vi "Teleop.vi"(10 "Match Info":T1={"Autonomous Elapsed Seconds"=0.0, "TeleOp Elapsed Seconds"=0.0, "Disabled Elapsed Seconds"=0.0, "Visited Autonomous"=FALSE, "Visited TeleOp"=FALSE, "Visited Disabled"=FALSE, "Autonomous Settings"={"Autonomous Style"=enum."Independent", "VI Refnum"=refnum}}, 11 "Call Context":T2) -> ()   [LabVIEW 2012]
doc: "This VI is called for each TeleOp packet received from the DS where the robot is not disabled. It is often used to read from the joysticks and update I/O or to update setpoints for timed control loops. It should complete and return within 20 milliseconds or it may miss DS packets."
uses:
  <vilib>/Rock Robotics/WPI/DriverStation/WPI_DriverStationDerivedRobotMode.ctl
  <vilib>/Rock Robotics/WPI/DriverStation/WPI_DriverStationMatch Info.ctl
  <vilib>/Rock Robotics/WPI/CAN/Jaguar/SubVIs/WPI_CANJaguar_StatusSelect.ctl
  <vilib>/Rock Robotics/WPI/DriverStation/DriverStationLCD/WPI_DriverStationLCDLCDLine.ctl
  <vilib>/Rock Robotics/WPI/Relay/WPI_RelayValue.ctl
  Robot Global Data.vi
  <vilib>/Rock Robotics/WPI/Joystick/WPI_JoystickGetSetRefNum.vi
  <vilib>/Rock Robotics/WPI/CAN/Jaguar/SubVIs/WPI_CANJaguar_StatusChannelSelect.ctl
  <vilib>/Rock Robotics/WPI/RobotDrive/WPI_RobotDriveMecanumDrive_Cartesian.vi
panel:
  in  "ShooterSpeed":dbl=1000.0
  in  "BallScrewPosition":dbl=0.55
  in  "Position":dbl
  # "KEEP BETWEEN 0.5 AND 0.6"
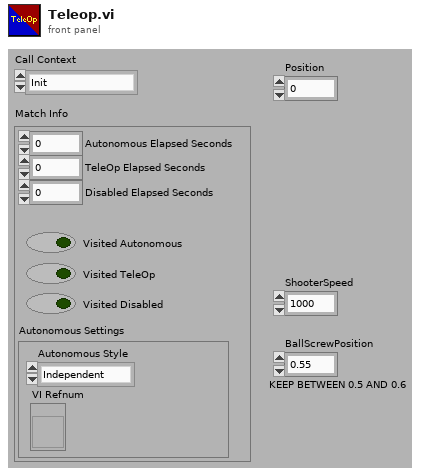
[diagram p1: front panel]
types:
  T1 = typedef "WPI_DriverStationMatch Info.ctl" = cluster{"Autonomous Elapsed Seconds":dbl, "TeleOp Elapsed Seconds":dbl, "Disabled Elapsed Seconds":dbl, "Visited Autonomous":bool, "Visited TeleOp":bool, "Visited Disabled":bool, "Autonomous Settings":cluster{"Autonomous Style":enum16{"Iterative", "Independent"}, "VI Refnum":refnum<vi>}}
  T2 = typedef "WPI_DriverStationDerivedRobotMode.ctl" = enum16{"Init", "Execute", "Stop"}
  T3 = typedef "WPI_DriverStationLCDLCDLine.ctl" = enum16{"Main - Line 1", "User - Line 2", "User - Line 3", "User - Line 4", "User - Line 5", "User - Line 6"}
  T4 = typedef "WPI_CANJaguar_StatusSelect.ctl" = enum16{"Output Percent VBus", "Output Voltage", "Bus Voltage", "Current", "Temperature", "Position", "Speed", "Limit Switches", "Faults", "Fault Counters", "Power Cycle"}
  T5 = cluster{bool, bool, bool, bool, bool, bool, i32, i32}
  T6 = typedef "WPI_JoystickDevRef.ctl" = cluster{"Device":T7}
  T7 = typedef "WPI_JoystickDeviceEnum.ctl" = enum16{"USB 1", "USB 2", "USB 3", "USB 4", "Kinect 1", "Kinect 2"}
  T8 = typedef "WPI_MotorControlDeviceRef.ctl" = cluster{"DeviceStatus":errorcluster, "Type":enum16{"PWM", "CAN"}, "PWM":cluster{"Digital Module":T9, "PWM Channel":T10, "DeadBand":T11}, "CAN":cluster{"Device Number":u8, "Control Mode":T12, "Semaphore":T13, "Max Vout":dbl}, "Invert":bool, "TransformRef":T14, "InvTransformRef":T14}
  T9 = typedef "FPGA_TypedefDigitalModule.ctl" = enum16{"Digital Module 1", "Digital Module 2"}
  T10 = typedef "FPGA_DIOPWMChannel.ctl" = enum8{"PWM 1", "PWM 2", "PWM 3", "PWM 4", "PWM 5", "PWM 6", "PWM 7", "PWM 8", "PWM 9", "PWM 10", "Invalid"}
  T11 = typedef "WPI_PWMDeadband.ctl" = cluster{"Name":string, "maxPositivePwm":i32, "minPositivePwm":i32, "centerPwm":i32, "maxNegativePwm":i32, "minNegativePwm":i32, "angularRange":u16}
  T12 = typedef "WPI_CANJaguar_ControlMode.ctl" = enum8{"Percent VBus", "Current", "Speed", "Position", "Voltage"}
  T13 = typedef "Semaphore RefNum" = refnum<k1>
  T14 = typedef "WPI_PWMTransform_ConPane.ctl" = refnum<vi>
  T15 = cluster{"Position":cluster{"X":dbl, "Y":dbl}, "Distance (ft)":dbl}
  T16 = typedef "WPI_DigitalInputDevRef.ctl" = cluster{"DevStatus":errorcluster, "DIO Channel":T17, "Digital Module":T9}
  T17 = typedef "FPGA_DIOChannel.ctl" = enum8{"DIO 1", "DIO 2", "DIO 3", "DIO 4", "DIO 5", "DIO 6", "DIO 7", "DIO 8", "DIO 9", "DIO 10", "DIO 11", "DIO 12", "DIO 13", "DIO 14", "Invalid"}
  T18 = typedef "WPI_RelayDevRef.ctl" = cluster{"DevStatus":errorcluster, "Relay Channel":T19, "Digital Module":T9, "Relay Direction":T20}
  T19 = typedef "FPGA_DIORelayChannel.ctl" = enum8{"Relay 1", "Relay 2", "Relay 3", "Relay 4", "Relay 5", "Relay 6", "Relay 7", "Relay 8", "Invalid"}
  T20 = typedef "WPI_RelayDirection.ctl" = enum16{"Both directions", "Forward only", "Reverse only"}
  T21 = typedef "WPI_CANJaguar_Status.ctl" = cluster{"Output Percent VBus":dbl, "Output Voltage":dbl, "Bus Voltage":dbl, "Current":dbl, "Temperature":dbl, "Position":dbl, "Speed":dbl, "Limits":cluster{"Forward Limit":bool, "Reverse Limit":bool, "Forward Soft Limit":bool, "Reverse Soft Limit":bool, "Sticky Forward Limit":bool, "Sticky Reverse Limit":bool, "Sticky Forward Soft Limit":bool, "Sticky Reverse Soft Limit":bool}, "Faults":cluster{"Current Fault":bool, "Temperature Fault":bool, "Bus Voltage Fault":bool, "Gate Driver Fault":bool, "Comm Fault":bool}, "Fault Counters":cluster{"Current Faults":u8, "Temperature Faults":u8, "Bus Voltage Faults":u8, "Gate Driver Faults":u8, "Comm Faults":u8, "CAN Status":u8, "CAN RX Errors":u8, "CAN TX Errors":u8}, "Power Cycle":bool}
  T22 = typedef "WPI_JoystickButtonState.ctl" = cluster{"Button 1":bool, "Button 2":bool, "Button 3":bool, "Button 4":bool, "Button 5":bool, "Button 6":bool, "Button 7":bool, "Button 8":bool, "Button 9":bool, "Button 10":bool, "Button 11":bool, "Button 12":bool}
  T23 = typedef "WPI_RelayValue.ctl" = enum16{"Off", "On", "Forward", "Reverse"}
  T24 = cluster{"axis 1 (x)":dbl, "axis 2 (y)":dbl, "axis 3 (throttle)":dbl, "axis 4":dbl, "axis 5":dbl, "axis 6":dbl}
  T25 = typedef "WPI_RobotDriveDevRef.ctl" = cluster{"DevStatus":errorcluster, "Motors[]":T8[], "Square Inputs":bool, "Max Output":dbl, "Isochronous":bool}
  T26 = typedef "WPI_CANJaguar_StatusChannelSelect.ctl" = enum16{"Periodic Status Channel 1", "Periodic Status Channel 2", "Periodic Status Channel 3", "Periodic Status Channel 4", "On Demand Status"}
  T27 = cluster{bool, bool, bool, bool, bool, bool, "DistanceOut":dbl, i32}
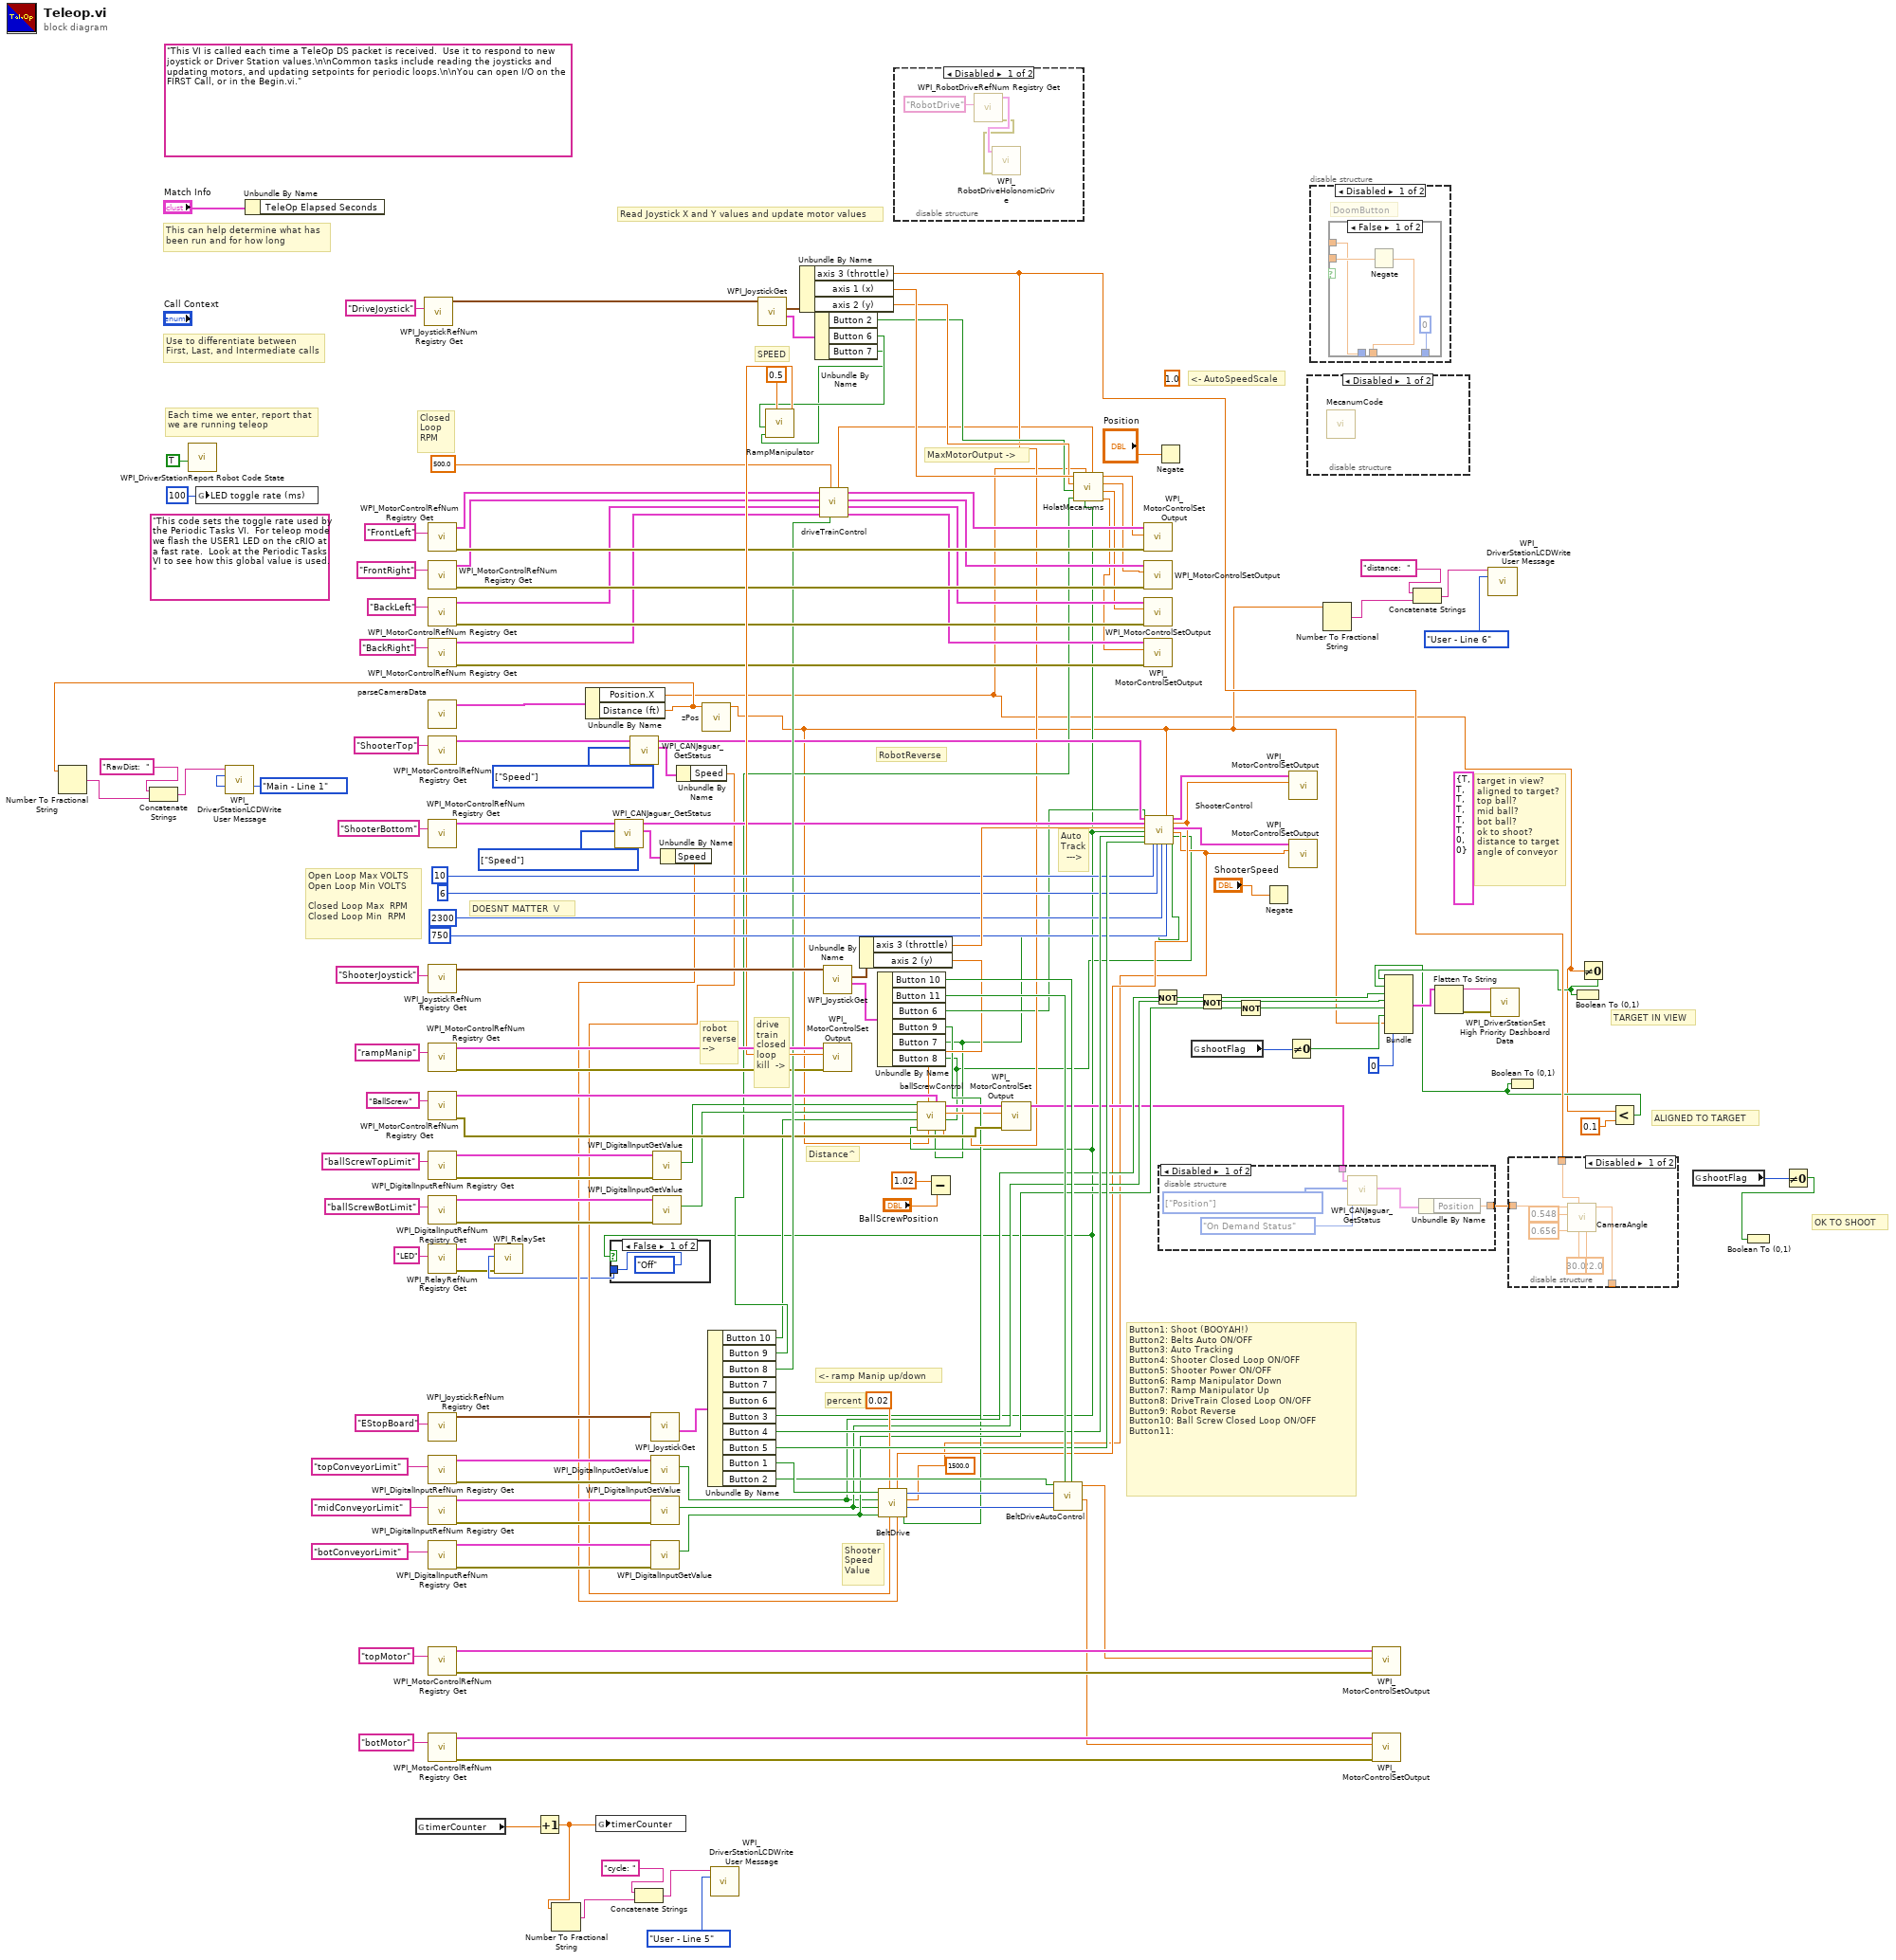
[diagram p0: block diagram]
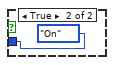
[diagram p3: hidden frame]
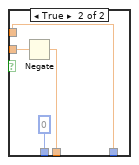
[diagram p5: hidden frame]
diagram:
  w74 = T4[] [enum."Speed"] items=["Output Percent VBus", "Output Voltage", "Bus Voltage", "Current", "Temperature", "Position", "Speed", "Limit Switches", "Faults", "Fault Counters", "Power Cycle"] ("Status Select")
  (unwired) T5 {TRUE, TRUE, TRUE, TRUE, TRUE, TRUE, 0, 0} ("AnalogModule[0]")
  (unwired) 1500.0 ("shootSpeedValue")
  w92 = T4[] [enum."Speed"] items=["Output Percent VBus", "Output Voltage", "Bus Voltage", "Current", "Temperature", "Position", "Speed", "Limit Switches", "Faults", "Fault Counters", "Power Cycle"] ("Status Select")
  (unwired) 1.0 ("CameraAutoSpeedScaler")
  (unwired) "This code sets the toggle rate used by the Periodic Tasks VI.  For teleop mode we flash the USER1 LED on the cRIO at a fast rate.  Look at the Periodic Tasks VI to see how this global value is used."
  (unwired) "This VI is called each time a TeleOp DS packet is received.  Use it to respond to new joystick or Driver Station values.\n\nCommon tasks include reading the joysticks and updating motors, and updating setpoints for periodic loops.\n\nYou can open I/O on the FIRST Call, or in the Begin.vi."
  # "ALIGNED TO TARGET"
  # "TARGET IN VIEW"
  # "OK TO SHOOT"
  # "DOESNT MATTER  \\/"
  # "Distance^"
  # "target in view?\naligned to target?\ntop ball?\nmid ball?\nbot ball?\nok to shoot?\ndistance to target\nangle of conveyor"
  # "Button1: Shoot (BOOYAH!)\nButton2: Belts Auto ON/OFF\nButton3: Auto Tracking\nButton4: Shooter Closed Loop ON/OFF\nButton5: Shooter Power ON/OFF\nButton6: Ramp Manipulator Down\nButton7: Ramp Manipulator Up\nButton8: DriveTrain Closed Loop ON/OFF\nButton9: Robot Reverse\nButton10: Ball Screw Closed Loop ON/OFF\nButton11:"
  # "SPEED"
  # "percent"
  # "Shooter\nSpeed\nValue"
  # "robot\nreverse\n-->"
  # "RobotReverse"
  # "Closed\nLoop\nRPM"
  # "<- ramp Manip up/down"
  # "drive\ntrain\nclosed\nloop\nkill  ->"
  # "MaxMotorOutput ->"
  # "<- AutoSpeedScale"
  # "Auto\nTrack\n  --->"
  # "Open Loop Max VOLTS\nOpen Loop Min VOLTS\n\nClosed Loop Max  RPM\nClosed Loop Min  RPM"
  # "Each time we enter, report that\nwe are running teleop"
  # "Use to differentiate between\nFirst, Last, and Intermediate calls"
  # "This can help determine what has\nbeen run and for how long"
  # "Read Joystick X and Y values and update motor values"
  n1 = call <vilib>:"WPI_DriverStationReport Robot Code State.vi"("TeleOp"=TRUE ("Autonomous")) -> ()  [unwired: 10 in, 1 out]
  n2 = global write "Robot Global Data.vi" "LED toggle rate (ms)"(u32 100 ("LED ms toggle rate")) -> ()
  n3 = Unbundle By Name("Match Info") -> ()  [unwired: 1 out]
  n4 = global read "Robot Global Data.vi" "timerCounter"() -> (w40:dbl)
  n5 = call <vilib>:"WPI_JoystickRefNum Registry Get.vi"("refnum name"="DriveJoystick") -> ("JoystickDevRef"=w157:T6)  [unwired: 9 in, 1 out]
  n6 = call <vilib>:"WPI_MotorControlRefNum Registry Get.vi"("refnum name"="FrontLeft") -> ("error out"=w105:errorcluster, "MotorControlDevRef"=w101:T8)  [unwired: 9 in]
  n7 = call <vilib>:"WPI_MotorControlRefNum Registry Get.vi"("refnum name"="FrontRight") -> ("error out"=w104:errorcluster, "MotorControlDevRef"=w100:T8)  [unwired: 9 in]
  n8 = call <vilib>:"WPI_MotorControlRefNum Registry Get.vi"("refnum name"="BackLeft") -> ("error out"=w103:errorcluster, "MotorControlDevRef"=w99:T8)  [unwired: 9 in]
  n9 = call <vilib>:"WPI_MotorControlRefNum Registry Get.vi"("refnum name"="BackRight") -> ("error out"=w102:errorcluster, "MotorControlDevRef"=w98:T8)  [unwired: 9 in]
  n10 = call "parseCameraData.vi"() -> ("TargetInfoOut"=w106:T15)  [unwired: 11 in]
  n11 = call <vilib>:"WPI_MotorControlRefNum Registry Get.vi"("refnum name"="ShooterTop") -> ("MotorControlDevRef"=w73:T8)  [unwired: 9 in, 1 out]
  n12 = call <vilib>:"WPI_MotorControlRefNum Registry Get.vi"("refnum name"="ShooterBottom") -> ("MotorControlDevRef"=w94:T8)  [unwired: 9 in, 1 out]
  n13 = call <vilib>:"WPI_JoystickRefNum Registry Get.vi"("refnum name"="ShooterJoystick") -> ("JoystickDevRef"=w147:T6)  [unwired: 9 in, 1 out]
  n14 = call <vilib>:"WPI_MotorControlRefNum Registry Get.vi"("refnum name"="rampManip") -> ("error out"=w87:errorcluster, "MotorControlDevRef"=w108:T8)  [unwired: 9 in]
  n15 = call <vilib>:"WPI_MotorControlRefNum Registry Get.vi"("refnum name"="BallScrew") -> ("error out"=w86:errorcluster, "MotorControlDevRef"=w89:T8)  [unwired: 9 in]
  n16 = call <vilib>:"WPI_DigitalInputRefNum Registry Get.vi"("refnum name"="ballScrewTopLimit") -> ("error out"=w83:errorcluster, "DigitalInputDevRef"=w82:T16)  [unwired: 9 in]
  n17 = call <vilib>:"WPI_DigitalInputRefNum Registry Get.vi"("refnum name"="ballScrewBotLimit") -> ("error out"=w84:errorcluster, "DigitalInputDevRef"=w85:T16)  [unwired: 9 in]
  n18 = call <vilib>:"WPI_RelayRefNum Registry Get.vi"("refnum name"="LED") -> ("error out"=w31:errorcluster, "RelayDevRef"=w34:T18)  [unwired: 9 in]
  n19 = call <vilib>:"WPI_JoystickRefNum Registry Get.vi"("refnum name"="EStopBoard") -> ("JoystickDevRef"=w127:T6)  [unwired: 9 in, 1 out]
  n20 = call <vilib>:"WPI_DigitalInputRefNum Registry Get.vi"("refnum name"="topConveyorLimit") -> ("error out"=w135:errorcluster, "DigitalInputDevRef"=w134:T16)  [unwired: 9 in]
  n21 = call <vilib>:"WPI_DigitalInputRefNum Registry Get.vi"("refnum name"="midConveyorLimit") -> ("error out"=w131:errorcluster, "DigitalInputDevRef"=w130:T16)  [unwired: 9 in]
  n22 = call <vilib>:"WPI_DigitalInputRefNum Registry Get.vi"("refnum name"="botConveyorLimit") -> ("error out"=w132:errorcluster, "DigitalInputDevRef"=w133:T16)  [unwired: 9 in]
  n23 = call <vilib>:"WPI_MotorControlRefNum Registry Get.vi"("refnum name"="topMotor") -> ("error out"=w137:errorcluster, "MotorControlDevRef"=w141:T8)  [unwired: 9 in]
  n24 = call <vilib>:"WPI_MotorControlRefNum Registry Get.vi"("refnum name"="botMotor") -> ("error out"=w136:errorcluster, "MotorControlDevRef"=w142:T8)  [unwired: 9 in]
  n25 = Increment(x=w40) -> (x+1=w17:dbl)
  n26 = Number To Fractional String(number=w17) -> (F-format string=w19:string)  [unwired: 3 in]
  n27 = Unbundle By Name(w106) -> ("Position.X"=w4:dbl, "Distance (ft)"=w16:dbl)
  n28 = Number To Fractional String(number=w16) -> (F-format string=w23:string)  [unwired: 3 in]
  n29 = Concatenate Strings("RawDist:  " ("line text"), w23) -> (w22:string)
  n30 = call <vilib>:"WPI_DriverStationLCDWrite User Message.vi"("line text"=w22, "line"=WPI_DriverStationLCDLCDLine."Main - Line 1") -> ()  [unwired: 13 in, 1 out]
  n31 = global write "Robot Global Data.vi" "timerCounter"(w17) -> ()
  n32 = call <vilib>:"WPI_CANJaguar_GetStatus.vi"("Status Select"=w92, "CAN Jaguar Ref"=w94) -> ("Status"=w91:T21, "CAN Jaguar Ref Out"=w93:T8)  [unwired: 7 in, 1 out]
  n33 = call <vilib>:"WPI_CANJaguar_GetStatus.vi"("Status Select"=w74, "CAN Jaguar Ref"=w73) -> ("Status"=w75:T21, "CAN Jaguar Ref Out"=w72:T8)  [unwired: 7 in, 1 out]
  n34 = Concatenate Strings("cycle: " ("line text"), w19) -> (w18:string)
  n35 = call <vilib>:"WPI_JoystickGet.vi"("JoystickDevRef"=w127) -> ("Buttons"=w128:T22)  [unwired: 4 in, 2 out]
  n36 = call <vilib>:"WPI_DigitalInputGetValue.vi"("error in (no error)"=w135, "DigitalInputDevRef"=w134) -> ("Value"=w54:bool)  [unwired: 7 in, 2 out]
  n37 = call <vilib>:"WPI_DigitalInputGetValue.vi"("error in (no error)"=w131, "DigitalInputDevRef"=w130) -> ("Value"=w55:bool)  [unwired: 7 in, 2 out]
  n38 = call <vilib>:"WPI_DigitalInputGetValue.vi"("error in (no error)"=w132, "DigitalInputDevRef"=w133) -> ("Value"=w68:bool)  [unwired: 7 in, 2 out]
  n39 = call <vilib>:"WPI_DigitalInputGetValue.vi"("error in (no error)"=w83, "DigitalInputDevRef"=w82) -> ("Value"=w79:bool)  [unwired: 7 in, 2 out]
  n40 = call <vilib>:"WPI_DigitalInputGetValue.vi"("error in (no error)"=w84, "DigitalInputDevRef"=w85) -> ("Value"=w78:bool)  [unwired: 7 in, 2 out]
  n41 = Unbundle By Name(w91) -> ("Speed"=w51:dbl)
  n42 = Unbundle By Name(w75) -> ("Speed"=w47:dbl)
  n43 = call "zPos.vi"("DistanceIn"=w16) -> ("DistanceOut"=w6:dbl)  [unwired: 10 in]
  n44 = Unbundle By Name(w128) -> ("Button 10"=w49:bool, "Button 9"=w56:bool, "Button 8"=w95:bool, "Button 3"=w33:bool, "Button 4"=w115:bool, "Button 5"=w114:bool, "Button 1"=w126:bool, "Button 2"=w123:bool)  [unwired: 2 out]
  n45 = case shown="False" w33 {
    tunnel: [WPI_RelayValue."Off" ("RelayValue") WPI_RelayValue."On" ("RelayValue")] -> w32
    frame False {
    }
    frame True {
    }
  }
  n46 = call <vilib>:"WPI_RelaySet.vi"("error in (no error)"=w31, "RelayValue"=w32, "RelayDevRef"=w34) -> ()  [unwired: 7 in, 2 out]
  n47 = call <vilib>:"WPI_DriverStationLCDWrite User Message.vi"("line text"=w18, "line"=WPI_DriverStationLCDLCDLine."User - Line 5") -> ()  [unwired: 13 in, 1 out]
  n48 = call <vilib>:"WPI_JoystickGet.vi"("JoystickDevRef"=w157) -> ("Buttons"=w155:T22, "Axes"=w156:T24)  [unwired: 4 in, 1 out]
  n49 = Unbundle By Name(w156) -> ("axis 3 (throttle)"=w50:dbl, "axis 1 (x)"=w59:dbl, "axis 2 (y)"=w58:dbl)
  n50 = Unbundle By Name(w155) -> ("Button 2"=w57:bool, "Button 6"=w2:bool, "Button 7"=w1:bool)
  n51 = call "RampManipulator.vi"("speed"=0.5, "rampManipDown"=w1, "rampManipUp"=w2) -> ("rampMotorValue"=w107:dbl)  [unwired: 8 in]
  n52 = call "driveTrainControl.vi"("driveTrainKillButton"=w95, "ClosedLoopMaxOutput"=500.0, "backRight"=w98, "backLeft"=w99, "frontRight"=w100, "frontLeft"=w101) -> ("backRight"=w69:T8, "backLeft"=w70:T8, "frontRight"=w97:T8, "frontLeft"=w71:T8, "drivetrainMaxOutput"=w48:dbl)  [unwired: 1 in]
  n53 = call <vilib>:"WPI_JoystickGet.vi"("JoystickDevRef"=w147) -> ("Buttons"=w148:T22, "Axes"=w149:T24)  [unwired: 4 in, 1 out]
  n54 = call <vilib>:"WPI_MotorControlSetOutput.vi"("error in (no error)"=w87, "Output"=w107, "MotorControlDevRef"=w108) -> ()  [unwired: 6 in, 3 out]
  n55 = Unbundle By Name(w149) -> ("axis 3 (throttle)"=w116:dbl, "axis 2 (y)"=w45:dbl)
  n56 = Unbundle By Name(w148) -> ("Button 10"=w121:bool, "Button 11"=w122:bool, "Button 6"=w46:bool, "Button 9"=w36:bool, "Button 7"=w5:bool, "Button 8"=w3:bool)
  n57 = disable-structure shown="Disabled" {
    frame Disabled {
      n58 = call <vilib>:"WPI_RobotDriveRefNum Registry Get.vi"("refnum name"="RobotDrive") -> ("error out"=w164:errorcluster, "RobotDriveDevRef"=w165:T25)  [unwired: 9 in]
      n59 = call-poly <vilib>:"WPI_RobotDriveHolonomicDrive.vi"("error in (no error)"=w164, "RobotDriveDevRef"=w165) -> ()  [unwired: 7 in, 3 out]
    }
    frame Enabled {
    }
  }
  n60 = call "ballScrewControl.vi"("joy1Wheel"=w50, "button8"=w3, "button7"=w5, "ballScrewMotorIN"=w89, "Distance"=w6, "joy2YAxis"=w45, "autoTrackingButton"=w33, "closedLoopKillButton"=w49, "ballScrewBotLimitSwitch"=w78, "ballScrewTopLimitSwitch"=w79) -> ("motorValueOutput"=w11:dbl, "ballScrewMotorOUT"=w88:T8)
  n61 = Subtract(x=1.02, y="BallScrewPosition") -> ()  [unwired: 1 out]
  n62 = call <vilib>:"WPI_MotorControlSetOutput.vi"("error in (no error)"=w86, "Output"=w11, "MotorControlDevRef"=w88) -> ("MotorControlDevRef"=w53:T8)  [unwired: 6 in, 2 out]
  n63 = call "HolatMecanums.vi"("MaxOutput"=w48, "AUTO TRACK BUTTON"=w33, "CAMERA X POS"=w4, "ROBOT REVERSE"=w56, "STRAFE BUTTON"=w57, "Y AXIS"=w58, "X AXIS"=w59) -> ("BackRight"=w29:dbl, "BackLeft"=w28:dbl, "FrontRight"=w27:dbl, "FrontLeft"=w26:dbl)  [unwired: 1 in]
  n64 = call <vilib>:"WPI_MotorControlSetOutput.vi"("error in (no error)"=w105, "Output"=w26, "MotorControlDevRef"=w71) -> ()  [unwired: 6 in, 3 out]
  n65 = call <vilib>:"WPI_MotorControlSetOutput.vi"("error in (no error)"=w104, "Output"=w27, "MotorControlDevRef"=w97) -> ()  [unwired: 6 in, 3 out]
  n66 = call <vilib>:"WPI_MotorControlSetOutput.vi"("error in (no error)"=w103, "Output"=w28, "MotorControlDevRef"=w70) -> ()  [unwired: 6 in, 3 out]
  n67 = call <vilib>:"WPI_MotorControlSetOutput.vi"("error in (no error)"=w102, "Output"=w29, "MotorControlDevRef"=w69) -> ()  [unwired: 6 in, 3 out]
  n68 = call "ShooterControl.vi"("ShooterTop"=w72, "ShooterBottom"=w93, "ThrottleAxis"=w116, "AutoTrack"=w33, "ClosedLoopKillSwitch"=w115, "ON/OFF"=w114, "OpenLoopMax"=10, "OpenLoopMin"=6, "button6"=w46, "ClosedLoopMax"=2300, "Distance"=w6, "ClosedLoopMin"=750, "button8"=w3, "button7"=w5) -> ("ShooterTop"=w118:T8, "ShooterTopValue"=w9:dbl, "ShooterBottom"=w117:T8, "ShooterBottomValue"=w8:dbl)  [unwired: 2 in]
  n69 = call "BeltDrive.vi"("button9"=w36, "shootSpeedValueBot"=w8, "encoderBottomFeedback"=w51, "shootSpeedValueTop"=w9, "encoderTopFeedback"=w47, "percent"=0.02, "botLimit"=w68, "midLimit"=w55, "topLimit"=w54, "shootButton"=w126) -> ("botMotor"=w125:i8, "topMotor"=w124:i8)
  n70 = call "BeltDriveAutoControl.vi"("Button 10"=w121, "Button 11"=w122, "botMotor"=w125, "topMotor"=w124, "BeltDriveAutoOnOff"=w123) -> ("botMotor"=w119:dbl, "topMotor"=w120:dbl)  [unwired: 5 in]
  n71 = Not(x=w54) -> (.not. x?=w64:bool)
  n72 = Negate(x="Position") -> ()  [unwired: 1 out]
  n73 = disable-structure shown="Disabled" {
    disable-tunnel: w53 -> [w168 _]
    disable-tunnel: [w167 _] -> w52
    frame Disabled {
      w170 = T4[] [enum."Position"] items=["Output Percent VBus", "Output Voltage", "Bus Voltage", "Current", "Temperature", "Position", "Speed", "Limit Switches", "Faults", "Fault Counters", "Power Cycle"] ("Status Select")
      n74 = call <vilib>:"WPI_CANJaguar_GetStatus.vi"("Status Channel Select"=WPI_CANJaguar_StatusChannelSelect."On Demand Status", "Status Select"=w170, "CAN Jaguar Ref"=w168) -> ("Status"=w171:T21)  [unwired: 6 in, 2 out]
      n75 = Unbundle By Name(w171) -> ("Position"=w167:dbl)
    }
    frame Enabled {
    }
  }
  n76 = global read "Robot Global Data.vi" "shootFlag"() -> (w61:u8)
  n77 = Not(x=w55) -> (.not. x?=w63:bool)
  n78 = Not(x=w68) -> (.not. x?=w62:bool)
  n79 = Negate(x="ShooterSpeed") -> ()  [unwired: 1 out]
  n80 = Not Equal To 0?(x=w61) -> (x != 0?=w65:bool)
  n81 = call <vilib>:"WPI_MotorControlSetOutput.vi"("Output"=w9, "MotorControlDevRef"=w118) -> ()  [unwired: 7 in, 3 out]
  n82 = call <vilib>:"WPI_MotorControlSetOutput.vi"("Output"=w8, "MotorControlDevRef"=w117) -> ()  [unwired: 7 in, 3 out]
  n83 = disable-structure shown="Disabled" {
    frame Disabled {
      n84 = call "MecanumCode.vi"() -> ()  [unwired: 8 in, 4 out]
    }
    frame Enabled {
    }
  }
  n85 = disable-structure shown="Disabled" {
    frame Disabled {
      # "DoomButton"
      n86 = case shown="False" {
        selector: _ -> [_ _]
        tunnel: [0 w178] -> _
        tunnel: [w173 w177] -> _
        tunnel: [w172 0] -> _
        tunnel: _ -> [w172 w178]
        tunnel: _ -> [w174 w176]
        frame False {
          n87 = Negate(x=w174) -> (-x=w173:dbl)
        }
        frame True {
          n88 = Negate(x=w176) -> (-x=w177:dbl)
        }
      }
    }
    frame Enabled {
    }
  }
  n89 = Number To Fractional String(number=w6) -> (F-format string=w42:string)  [unwired: 3 in]
  n90 = call <vilib>:"WPI_MotorControlSetOutput.vi"("error in (no error)"=w137, "Output"=w120, "MotorControlDevRef"=w141) -> ()  [unwired: 6 in, 3 out]
  n91 = call <vilib>:"WPI_MotorControlSetOutput.vi"("error in (no error)"=w136, "Output"=w119, "MotorControlDevRef"=w142) -> ()  [unwired: 6 in, 3 out]
  n92 = Concatenate Strings("distance:  " ("line text"), w42) -> (w41:string)
  n93 = call <vilib>:"WPI_DriverStationLCDWrite User Message.vi"("line text"=w41, "line"=WPI_DriverStationLCDLCDLine."User - Line 6") -> ()  [unwired: 13 in, 1 out]
  n94 = disable-structure shown="Disabled" {
    disable-tunnel: w52 -> [w186 _]
    disable-tunnel: w50 -> [w183 _]
    disable-tunnel: [w180 _] -> _
    frame Disabled {
      n95 = call "CameraAngle.vi"("MinAngle"=22.0, "MaxAngle"=30.0, "joystickWheel"=w183, "POT VALUE AT 80*"=0.656, "POT VALUE AT 50*"=0.548, "Pot Value"=w186) -> ("ServoAngle"=w180:dbl)  [unwired: 5 in]
    }
    frame Enabled {
    }
  }
  n96 = Not Equal To 0?(x=w4) -> (x != 0?=w15:bool)
  n97 = Boolean To (0,1)(Boolean=w15) -> ()  [unwired: 1 out]
  n98 = Less?(x=w4, y=0.1) -> (x < y?=w14:bool)
  n99 = Bundle(w15, w14, w64, w63, w62, w65, "DistanceOut"=w6, 0) -> (w66:T27)  [unwired: 1 in]
  n100 = Flatten To String(anything=w66) -> (data string=w67:string, error out=w7:errorcluster)  [unwired: 3 in, 1 out]
  n101 = call <vilib>:"WPI_DriverStationSet High Priority Dashboard Data.vi"("error in (no error)"=w7, "User Data"=w67) -> ()  [unwired: 9 in, 1 out]
  n102 = Boolean To (0,1)(Boolean=w14) -> ()  [unwired: 1 out]
  n103 = global read "Robot Global Data.vi" "shootFlag"() -> (w38:u8)
  n104 = Not Equal To 0?(x=w38) -> (x != 0?=w37:bool)
  n105 = Boolean To (0,1)(Boolean=w37) -> ()  [unwired: 1 out]
